vi "DeletedCommunity.vi"(11 "ProgramData":T1) -> (3 "ReturnedStates":enum16{"DeleteConfirmed", "CancelDelete"}(ring)=enum."CancelDelete")   [LabVIEW 2019]
uses:
  ProductsCluster.ctl
  ReturnedValues.ctl
panel:
  in  "Cancel Button":bool
  in  "OK Button":bool
  out "Usuniêty Produkt":T1
  # "Czy na pewno chcesz usun¹æ z bazy \n      danych  nastêpuj¹cy produkt:"
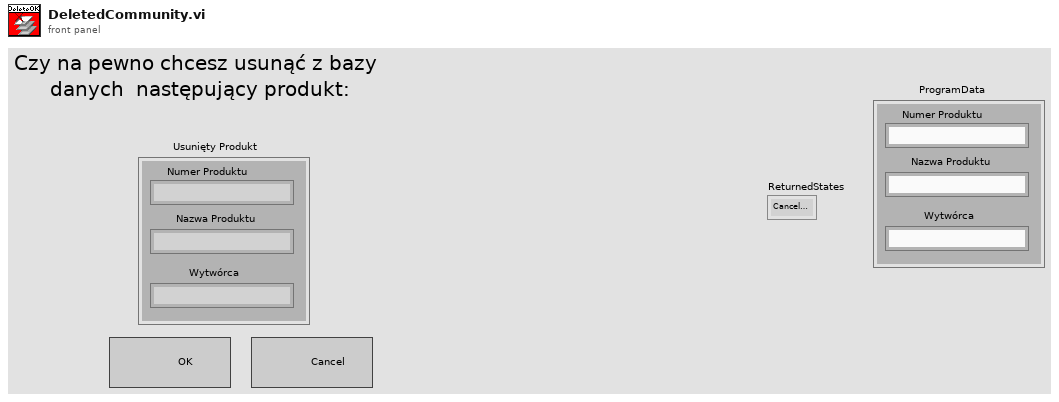
[diagram p1: front panel]
types:
  T1 = typedef "ProductsCluster.ctl" = cluster{"Numer Produktu":string, "Nazwa Produktu":string, "Wytwórca":string}
  T2 = typedef "ReturnedValues.ctl" = enum16{"DeleteConfirmed", "CancelDelete"}
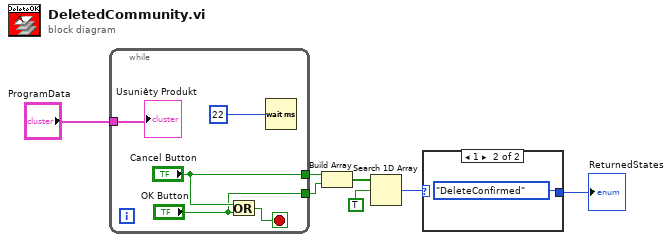
[diagram p0: block diagram]
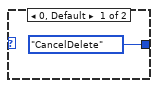
[diagram p2: hidden frame]
diagram:
  n1 = while {
    tunnel: "ProgramData" -> [w12]
    tunnel: ["Cancel Button"] -> w5
    tunnel: ["OK Button"] -> w6
    stop <- w10 stop-if-true
    n2 = Or(x="Cancel Button", y="OK Button") -> (x .or. y?=w10:bool)
    n3 = Wait (ms)(milliseconds to wait=u32 22) -> ()  [unwired: 1 out]
    "Usuniêty Produkt" <- w12
  }
  n4 = Build Array(w5, w6) -> (w4:bool[])
  n5 = Search 1D Array(1D array=w4, element=TRUE) -> (index of element=w2:i32)  [unwired: 1 in]
  n6 = case shown="1" w2 {
    tunnel: [ReturnedValues."CancelDelete" ("ReturnedStates") ReturnedValues."DeleteConfirmed" ("ReturnedStates")] -> w1
    frame 0, Default {
    }
    frame 1 {
    }
  }
  "ReturnedStates" <- w1
